vi "Read Instances.vi"(8 "error in (no error)":errorcluster, 11 "Polynomial in":refnum<class "Polynomial.lvclass">) -> (0 "error out":errorcluster, 2 "Scaling Instances":string[](array[string]), 3 "Polynomial in":refnum<class "Polynomial.lvclass">)   [LabVIEW 2018, in "Polynomial.lvclass"]
doc: "Polynomial.lvclass:Read Instances.vi\n\nThis VI assembles a list of all the names of Polynomials defined in the current configuration file.\n\nInstrument Communication Module Version 1.0\nSeptember, 2017 Original Code Consulting David Thomson\n www.originalcode.com"
uses:
  Polynomial.lvclass
  Polynomial.lvclass/Polynomial.ctl
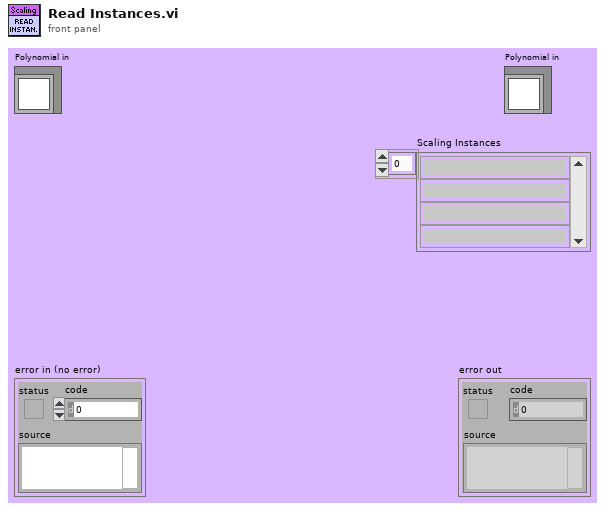
[diagram p1: front panel]
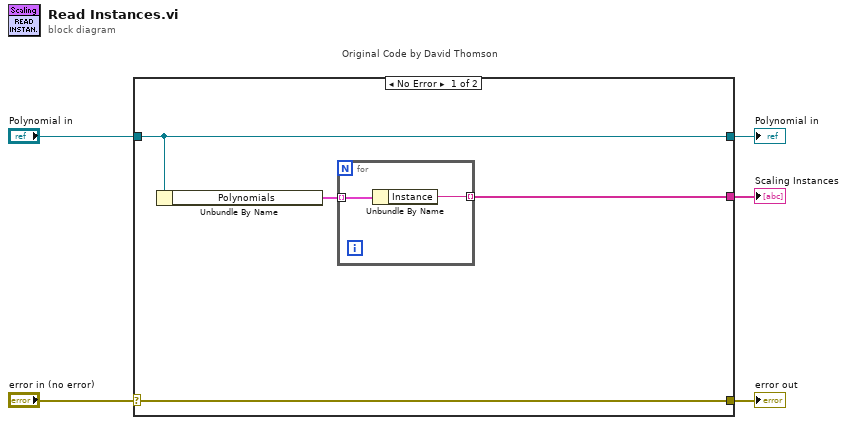
[diagram p0: block diagram]
diagram:
  n1 = case "Original Code by David Thomson" shown="No Error" "error in (no error)" {
    selector: "error in (no error)" -> [w9 w13]
    tunnel: [w9 w13] -> w4
    tunnel: [w8 w12] -> w2
    tunnel: "Polynomial in" -> [w8 w12]
    tunnel: [w6 _] -> w1
    frame No Error {
      n2 = Unbundle By Name(w8) -> ("Polynomials"=w7:cluster{"Instance":string, "Polynomial":dbl[]}[])
      n3 = for {
        tunnel: w7 -> [w11] mode=indexing
        tunnel: [w10] -> w6 mode=indexing
        n4 = Unbundle By Name(w11) -> ("Instance"=w10:string)
      }
    }
    frame Error {
    }
  }
  "error out" <- w4
  "Polynomial in" <- w2
  "Scaling Instances" <- w1
